vi "BuildTagString.vi"(8 "byte order":T1(ring)=enum."little-endian", 10 "Tag":T3={"Data Type"=enum."miUINT32", "# bytes"=8, "data"="\u0006\f\u0000\u0000\u0000\u0000\u0000\u0000"}, 11 "String In":string) -> (1 "Compressed String Out":string, 3 "String Out":string)   [LabVIEW 2022 SP3]
uses:
  miDataType.ctl
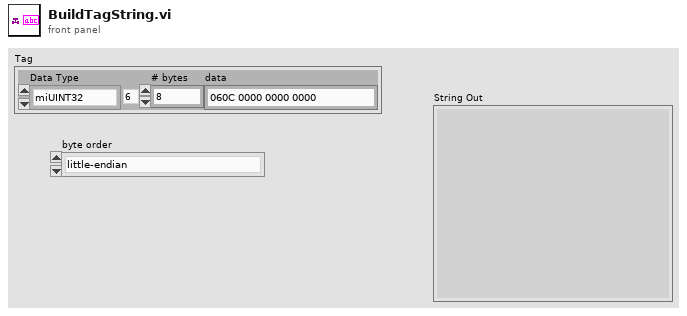
[diagram p1: front panel]
types:
  T1 = enum16{"big-endian, network order", "native, host order", "little-endian"}
  T2 = typedef "miDataType.ctl" = enum16{"illegal", "miINT8", "miUINT8", "miINT16", "miUINT16", "miINT32", "miUINT32", "miSINGLE", "--", "miDOUBLE", "---", "----", "miINT64", "miUINT64", "miMATRIX", "miCOMPRESSED", "miUTF8", "miUTF16", "miUTF32", "udefined"}
  T3 = cluster{"Data Type":T2, "# bytes":u32, "data":string}
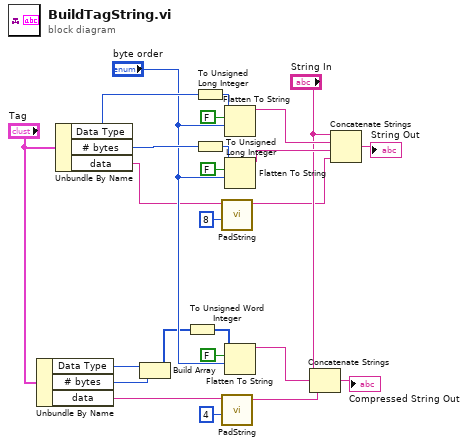
[diagram p0: block diagram]
diagram:
  n1 = Unbundle By Name("Tag") -> ("Data Type"=w10:T2, "# bytes"=w8:u32, "data"=w3:string)
  n2 = Unbundle By Name("Tag") -> ("Data Type"=w23:T2, "# bytes"=w20:u32, "data"=w6:string)
  n3 = Build Array(w10, w8) -> (w9:u32[])
  n4 = To Unsigned Word Integer(number=w9) -> (unsigned 16bit integer=w15:u16[])
  n5 = To Unsigned Long Integer(number=w23) -> (unsigned 32bit integer=w24:u32)
  n6 = To Unsigned Long Integer(number=w20) -> (unsigned 32bit integer=w22:u32)
  n7 = call "PadString.vi"("size"=8, "data"=w6) -> ("String"=w5:string)  [unwired: 9 in]
  n8 = call "PadString.vi"("size"=4, "data"=w3) -> ("String"=w1:string)  [unwired: 9 in]
  n9 = Flatten To String(anything=w24, prepend array or string size? (T)=FALSE ("data includes array or string size? (T)"), byte order (0:big-endian, network order)="byte order") -> (data string=w19:string)  [unwired: 1 in, 2 out]
  n10 = Flatten To String(anything=w22, prepend array or string size? (T)=FALSE ("data includes array or string size? (T)"), byte order (0:big-endian, network order)="byte order") -> (data string=w18:string)  [unwired: 1 in, 2 out]
  n11 = Flatten To String(anything=w15, prepend array or string size? (T)=FALSE ("data includes array or string size? (T)"), byte order (0:big-endian, network order)="byte order") -> (data string=w16:string)  [unwired: 1 in, 2 out]
  n12 = Concatenate Strings("String In", w16, w1) -> (→"Compressed String Out":string)
  n13 = Concatenate Strings("String In", w19, w18, w5) -> (→"String Out":string)
